vi "SCS Main.vi"() -> ()   [LabVIEW 2016]
doc: "Use this template to build a simple state machine design pattern. Each state executes code and determines which state to transition to."
uses:
  controls/SCS State.ctl
  controls/SCS Data.ctl
panel:
  in  "Solar Cell Stand Control":T1(tab)
  in  "NI Elvis Board":tag
  in  "Start Voltage, V:":dbl caption="MOSFET Control Voltage Range, V:"
  in  "Stop Voltage, V:":dbl=-10.0
  in  "Step Voltage, V:":dbl=0.1
  in  "Measurement pause, ms:":u32=250
  in  "Area of Solar Cell, m^2:":dbl=0.1
  in  "Light Intensity/ Irradiance, W/m^2:":dbl(knob)=600.0 scale=0.0..1200.0
  in  "Data from file":bool
  in  "Measure I-V Curve":bool
  out "Progress":u8(slide) max=100 scale=0.0..100.0
  out "Current (Amps) vs Voltage (Volts)":cluster{"voltage":dbl[], "current":dbl[]}(graph)
  in  "Voltage Data":path=path "E:/UPWORK/solar/labview/003/SolarCellStand/Sample Data/voltage - foward - bias - 001.lvm" caption="File Name"
  in  "Current Data":path=path "E:/UPWORK/solar/labview/003/SolarCellStand/Sample Data/current - foward - bias - 001.lvm" caption="File Name"
  in  "Calculate Solar Cell Parameters":bool
  out "Short Circuit Current Isc, A:":dbl format="%.5f"
  out "Open Circuit Voltage Voc, V:":dbl format="%.5f"
  out "Efficiency, %:":dbl format="%.5f"
  out "Fill Factor:":dbl format="%.5f"
  out "Pmax, W:":dbl format="%.5f"
  out "Voltage at Pmax, V:":dbl format="%.5f"
  out "Current at Pmax, A:":dbl format="%.5f"
  out "Current and Power vs. Voltage":cluster{"voltage":dbl[], "current":dbl[]}[](graph)=[{"voltage"=[0.00134, 0.011411, 0.025834, 0.043904, 0.055853, 0.075347, 0.099155, 0.125663, 0.165263, 0.217428, 0.267874, 0.315752, 0.36725, 0.425099, 0.474937, 0.530085, 0.588472, 0.643221, 0.694358, 0.754622, 0.812053, 0.873564, 0.938448, 0.995444, 1.055319, 1.116484, 1.181096, 1.242979, 1.310054, 1.384923, 1.457974, 1.528483, 1.591961, 1.655914, 1.723383, 1.78537, 1.841803, 1.874735, 1.918172, 1.968127, 2.017264, 2.064175, 2.116398, 2.158177, 2.191225, 2.218755, 2.24048, 2.261856, 2.280808, 2.297463, 2.312474, 2.325391, 2.338537, 2.350645, 2.362017, 2.372641, 2.381227, 2.390448, 2.39921, 2.407016, 2.414358, 2.421423, 2.428593, 2.435115, 2.441853, 2.447216, 2.45325, 2.459011, 2.464522, 2.470157, 2.474042, 2.47733, 2.481663, 2.486527, 2.491175, 2.496801, 2.501739, 2.507229, 2.511954, 2.515881, 2.519776, 2.523798, 2.526966, 2.530482, 2.534179, 2.537454, 2.540996, 2.544249, 2.547457, 2.550411, 2.553712, 2.556938, 2.559943, 2.562754, 2.565624, 2.568656, 2.571368, 2.573971, 2.576844, 2.579394, 2.581922, 2.584569, 2.58696, 2.589667, 2.592003, 2.594428, 2.596938, 2.59895, 2.601485, 2.603775, 2.606028, 2.608198, 2.610307, 2.6125, 2.614489, 2.616517, 2.618693, 2.620546, 2.622788, 2.624713, 2.626775, 2.628652, 2.630374, 2.632358, 2.634291, 2.635909, 2.637872, 2.639706, 2.6416, 2.64327, 2.64507, 2.646937, 2.64855, 2.650292, 2.651969, 2.653556, 2.655158, 2.656701, 2.658523, 2.66009, 2.661507, 2.663332, 2.664731, 2.666314, 2.667904, 2.669272, 2.67096, 2.672271, 2.67381, 2.675234, 2.676598, 2.67819, 2.679489, 2.681023, 2.682384, 2.683646, 2.68527, 2.686444, 2.688037, 2.689359, 2.69057, 2.692017, 2.693188, 2.694379, 2.695854, 2.697093, 2.698419, 2.699635, 2.700981, 2.702147, 2.703366, 2.704606, 2.705739, 2.707068, 2.708254, 2.70947, 2.710647, 2.711858, 2.713057, 2.714301, 2.71546, 2.716741, 2.717737, 2.719024, 2.720152, 2.72107, 2.722252, 2.723341, 2.724516, 2.725631, 2.726557, 2.727808, 2.728738, 2.72989, 2.731069, 2.732, 2.733089, 2.734104, 2.73519, 2.736257, 2.737217, 2.738296, 2.739307, 2.740423, 2.741454, 2.742348, 2.743357, 2.744268, 2.745417, 2.746408, 2.747273, 2.74838, 2.749326, 2.750382, 2.751351, 2.752211, 2.753257, 2.754209, 2.755152, 2.756018, 2.756854, 2.757837, 2.758826, 2.759727, 2.760683, 2.761421, 2.76238, 2.763236, 2.764109, 2.764945, 2.76579, 2.76688, 2.767667, 2.768646, 2.769522, 2.770365, 2.771362, 2.772145, 2.773009, 2.7739, 2.774781, 2.775641, 2.776447, 2.777355, 2.778196, 2.778952, 2.779808], "current"=[0.11683, 0.116793, 0.116696, 0.116612, 0.116353, 0.116156, 0.115983, 0.115806, 0.115674, 0.115608, 0.115475, 0.115277, 0.115048, 0.114847, 0.114559, 0.114304, 0.114054, 0.113759, 0.113435, 0.11314, 0.112824, 0.112487, 0.112162, 0.111794, 0.111412, 0.111022, 0.11061, 0.110173, 0.109698, 0.109199, 0.108699, 0.1082, 0.107699, 0.107197, 0.106697, 0.106198, 0.105698, 0.105198, 0.104695, 0.104194, 0.103695, 0.103195, 0.102695, 0.102193, 0.101693, 0.101194, 0.100694, 0.10019, 0.09969, 0.09919, 0.098688, 0.098188, 0.097687, 0.097188, 0.096685, 0.096185, 0.095685, 0.095182, 0.094683, 0.094182, 0.093684, 0.093181, 0.092681, 0.09218, 0.091678, 0.091179, 0.090679, 0.090175, 0.089677, 0.089173, 0.088675, 0.088175, 0.087671, 0.087173, 0.086673, 0.086171, 0.085671, 0.085168, 0.08467, 0.08417, 0.083668, 0.083169, 0.082665, 0.082166, 0.081662, 0.081164, 0.080665, 0.080162, 0.079663, 0.079161, 0.07866, 0.078158, 0.077659, 0.077157, 0.076657, 0.076154, 0.075655, 0.075152, 0.074654, 0.074151, 0.073652, 0.07315, 0.07265, 0.072148, 0.071649, 0.071146, 0.070648, 0.070145, 0.069642, 0.069142, 0.068641, 0.068141, 0.067638, 0.067141, 0.066638, 0.066136, 0.065636, 0.065134, 0.064635, 0.064133, 0.063635, 0.063132, 0.062629, 0.06213, 0.061629, 0.061126, 0.060626, 0.060125, 0.059626, 0.059125, 0.058622, 0.058124, 0.057621, 0.057119, 0.056621, 0.056118, 0.055616, 0.055117, 0.054616, 0.054112, 0.053614, 0.053113, 0.05261, 0.052112, 0.051611, 0.051108, 0.05061, 0.050108, 0.049607, 0.049108, 0.048606, 0.048102, 0.047606, 0.047103, 0.046601, 0.046103, 0.045601, 0.045099, 0.044597, 0.044099, 0.043596, 0.043094, 0.042597, 0.042095, 0.041591, 0.041095, 0.040592, 0.040089, 0.039591, 0.03909, 0.038588, 0.038087, 0.037589, 0.037087, 0.036585, 0.036086, 0.035586, 0.035083, 0.034584, 0.034083, 0.033583, 0.033083, 0.032581, 0.03208, 0.031582, 0.03108, 0.030583, 0.030082, 0.029579, 0.02908, 0.02858, 0.028078, 0.02758, 0.02708, 0.026582, 0.026079, 0.025578, 0.025081, 0.02458, 0.02408, 0.02358, 0.023082, 0.02258, 0.022079, 0.021581, 0.021081, 0.020581, 0.020081, 0.019536, 0.019036, 0.018535, 0.018034, 0.017533, 0.017033, 0.016532, 0.016031, 0.01553, 0.01503, 0.014529, 0.014028, 0.013528, 0.013027, 0.012526, 0.012026, 0.011525, 0.011024, 0.010524, 0.010023, 0.009523, 0.009022, 0.008521, 0.00802, 0.007519, 0.007018, 0.006517, 0.006016, 0.005515, 0.005015, 0.004514, 0.004013, 0.003512, 0.003012, 0.002512, 0.002012, 0.001507, 0.001006, 0.000505]}, {"voltage"=[0.00134, 0.011411, 0.025834, 0.043904, 0.055853, 0.075347, 0.099155, 0.125663, 0.165263, 0.217428, 0.267874, 0.315752, 0.36725, 0.425099, 0.474937, 0.530085, 0.588472, 0.643221, 0.694358, 0.754622, 0.812053, 0.873564, 0.938448, 0.995444, 1.055319, 1.116484, 1.181096, 1.242979, 1.310054, 1.384923, 1.457974, 1.528483, 1.591961, 1.655914, 1.723383, 1.78537, 1.841803, 1.874735, 1.918172, 1.968127, 2.017264, 2.064175, 2.116398, 2.158177, 2.191225, 2.218755, 2.24048, 2.261856, 2.280808, 2.297463, 2.312474, 2.325391, 2.338537, 2.350645, 2.362017, 2.372641, 2.381227, 2.390448, 2.39921, 2.407016, 2.414358, 2.421423, 2.428593, 2.435115, 2.441853, 2.447216, 2.45325, 2.459011, 2.464522, 2.470157, 2.474042, 2.47733, 2.481663, 2.486527, 2.491175, 2.496801, 2.501739, 2.507229, 2.511954, 2.515881, 2.519776, 2.523798, 2.526966, 2.530482, 2.534179, 2.537454, 2.540996, 2.544249, 2.547457, 2.550411, 2.553712, 2.556938, 2.559943, 2.562754, 2.565624, 2.568656, 2.571368, 2.573971, 2.576844, 2.579394, 2.581922, 2.584569, 2.58696, 2.589667, 2.592003, 2.594428, 2.596938, 2.59895, 2.601485, 2.603775, 2.606028, 2.608198, 2.610307, 2.6125, 2.614489, 2.616517, 2.618693, 2.620546, 2.622788, 2.624713, 2.626775, 2.628652, 2.630374, 2.632358, 2.634291, 2.635909, 2.637872, 2.639706, 2.6416, 2.64327, 2.64507, 2.646937, 2.64855, 2.650292, 2.651969, 2.653556, 2.655158, 2.656701, 2.658523, 2.66009, 2.661507, 2.663332, 2.664731, 2.666314, 2.667904, 2.669272, 2.67096, 2.672271, 2.67381, 2.675234, 2.676598, 2.67819, 2.679489, 2.681023, 2.682384, 2.683646, 2.68527, 2.686444, 2.688037, 2.689359, 2.69057, 2.692017, 2.693188, 2.694379, 2.695854, 2.697093, 2.698419, 2.699635, 2.700981, 2.702147, 2.703366, 2.704606, 2.705739, 2.707068, 2.708254, 2.70947, 2.710647, 2.711858, 2.713057, 2.714301, 2.71546, 2.716741, 2.717737, 2.719024, 2.720152, 2.72107, 2.722252, 2.723341, 2.724516, 2.725631, 2.726557, 2.727808, 2.728738, 2.72989, 2.731069, 2.732, 2.733089, 2.734104, 2.73519, 2.736257, 2.737217, 2.738296, 2.739307, 2.740423, 2.741454, 2.742348, 2.743357, 2.744268, 2.745417, 2.746408, 2.747273, 2.74838, 2.749326, 2.750382, 2.751351, 2.752211, 2.753257, 2.754209, 2.755152, 2.756018, 2.756854, 2.757837, 2.758826, 2.759727, 2.760683, 2.761421, 2.76238, 2.763236, 2.764109, 2.764945, 2.76579, 2.76688, 2.767667, 2.768646, 2.769522, 2.770365, 2.771362, 2.772145, 2.773009, 2.7739, 2.774781, 2.775641, 2.776447, 2.777355, 2.778196, 2.778952, 2.779808], "current"=[0.0001565522, 0.0013327249229999998, 0.0030147244639999998, 0.0051197332479999995, 0.0064986641089999995, 0.008752006132, 0.011500294365, 0.014552529378000001, 0.019116632262, 0.025136416224, 0.030932750149999997, 0.036398943304, 0.042251378, 0.048821344853, 0.054408307782999994, 0.06059083584, 0.067117585488, 0.073172177739, 0.07876449972999999, 0.08537793308000001, 0.091619067672, 0.098264593668, 0.10525820457599999, 0.111284666536, 0.11757520042799999, 0.123954286648, 0.13064102855999998, 0.136942725367, 0.14371030369200002, 0.151232206677, 0.15848031582600003, 0.1653818606, 0.171452607739, 0.17750901305800001, 0.183879795951, 0.18960272326, 0.194674893494, 0.19721837253, 0.20082301753999998, 0.20506702463799997, 0.20918019047999997, 0.213012539125, 0.21734349260999997, 0.220550582161, 0.22283224392500003, 0.22452469346999998, 0.22560289311999998, 0.22661535264, 0.22737374952, 0.22788535497, 0.22821343411199999, 0.22832549150800002, 0.228444663919, 0.22845448626, 0.22837161364499997, 0.228212474585, 0.22784770549500002, 0.227527621536, 0.22716440043000002, 0.226697580912, 0.226186714872, 0.22563061656299999, 0.22508442783299998, 0.2244689007, 0.22386419933399998, 0.223134707664, 0.22245825675, 0.221741316925, 0.22101093939400002, 0.220271310161, 0.21938567435, 0.21843857275, 0.217569876873, 0.21675801817100002, 0.21591761077500002, 0.215151838971, 0.214326481869, 0.213535679472, 0.21268714517999998, 0.21176170376999998, 0.210824618368, 0.20990175586200002, 0.20889164439, 0.20791958401200003, 0.20694612549799998, 0.205949916456, 0.20496944233999997, 0.20395208833800002, 0.202938066991, 0.201893085171, 0.20087498591999997, 0.19984516020400003, 0.198802613437, 0.19773441037800002, 0.196673038968, 0.19561342902399997, 0.19453684604000002, 0.19343906859199997, 0.19237171197599998, 0.191264644494, 0.190163719144, 0.18906122235000003, 0.18794264400000002, 0.186839294716, 0.18571442294700002, 0.18458317448800002, 0.18346847582400003, 0.18230334774999998, 0.18117261836999998, 0.18003021105, 0.17888036794799997, 0.17772521991799997, 0.17655594486600001, 0.1754058625, 0.174224317982, 0.173045968312, 0.171880533748, 0.170686643164, 0.16952390237999998, 0.16833071882899997, 0.167154827125, 0.16595205806399999, 0.16473769324600002, 0.16354840254, 0.16234872003900003, 0.161122573534, 0.159923627872, 0.15871232324999998, 0.15750804159999998, 0.15628333874999997, 0.15505929354, 0.153850566188, 0.15261209955000002, 0.151382028748, 0.15015713674899997, 0.148912255608, 0.147669267328, 0.146429389017, 0.145197892168, 0.14394279008, 0.142694036298, 0.141457552516, 0.14019149791, 0.13894695516799999, 0.137693193344, 0.136421153376, 0.1351772856, 0.13390215526799998, 0.13263969267, 0.131375391272, 0.130098722388, 0.12882629537999998, 0.127559753334, 0.126284226369, 0.12500177678399998, 0.12372413153799999, 0.12245099727000001, 0.12115593795599999, 0.11987838608899999, 0.118598042541, 0.11729808972000001, 0.11600978059799999, 0.11472172923600002, 0.113419884005, 0.11212326371400001, 0.110837036835, 0.109534224048, 0.10822566751499998, 0.10693453877100001, 0.10562692623, 0.10431748720799999, 0.10301032872200001, 0.10170602327099999, 0.10039703091600001, 0.09908147259000001, 0.09777393442, 0.096461084142, 0.09514011421400001, 0.093828363288, 0.092511520983, 0.09119329318000001, 0.089877942503, 0.088546589197, 0.08722628991999999, 0.085907840464, 0.08457085560000001, 0.08325463291600001, 0.08192354396200001, 0.080588458764, 0.07926134948, 0.07792499906000001, 0.07659139302399999, 0.07525859404, 0.07392542120000001, 0.072597276158, 0.07124782800000001, 0.069906950442, 0.06857406242399999, 0.0672309702, 0.06588906856, 0.06454357686, 0.063205348272, 0.061853552060000004, 0.060505799417, 0.059163318774, 0.05781143818799999, 0.056461030417, 0.055107645708, 0.05363446651200001, 0.052280622688, 0.050920705054999994, 0.04956428492000001, 0.048203932758, 0.046847256606, 0.045485334732000005, 0.044120694541, 0.04275808121, 0.04139576127, 0.040029603408, 0.038661420504, 0.037294720912, 0.035926342599, 0.034557054476, 0.033188476902, 0.031816871575, 0.030441905104, 0.02907128712, 0.027695914428000002, 0.026322610007, 0.024945333790000003, 0.02356729659, 0.0221903776, 0.020810088172999997, 0.019430357627999998, 0.018048974874, 0.01666651584, 0.015284061429999999, 0.013902307175000002, 0.012517362625999999, 0.011131660699999999, 0.009745030872, 0.008360230691999999, 0.006974434864, 0.00558803826, 0.004186741372, 0.0027956257119999997, 0.0014038030400000002]}]
  in  "Exit":bool
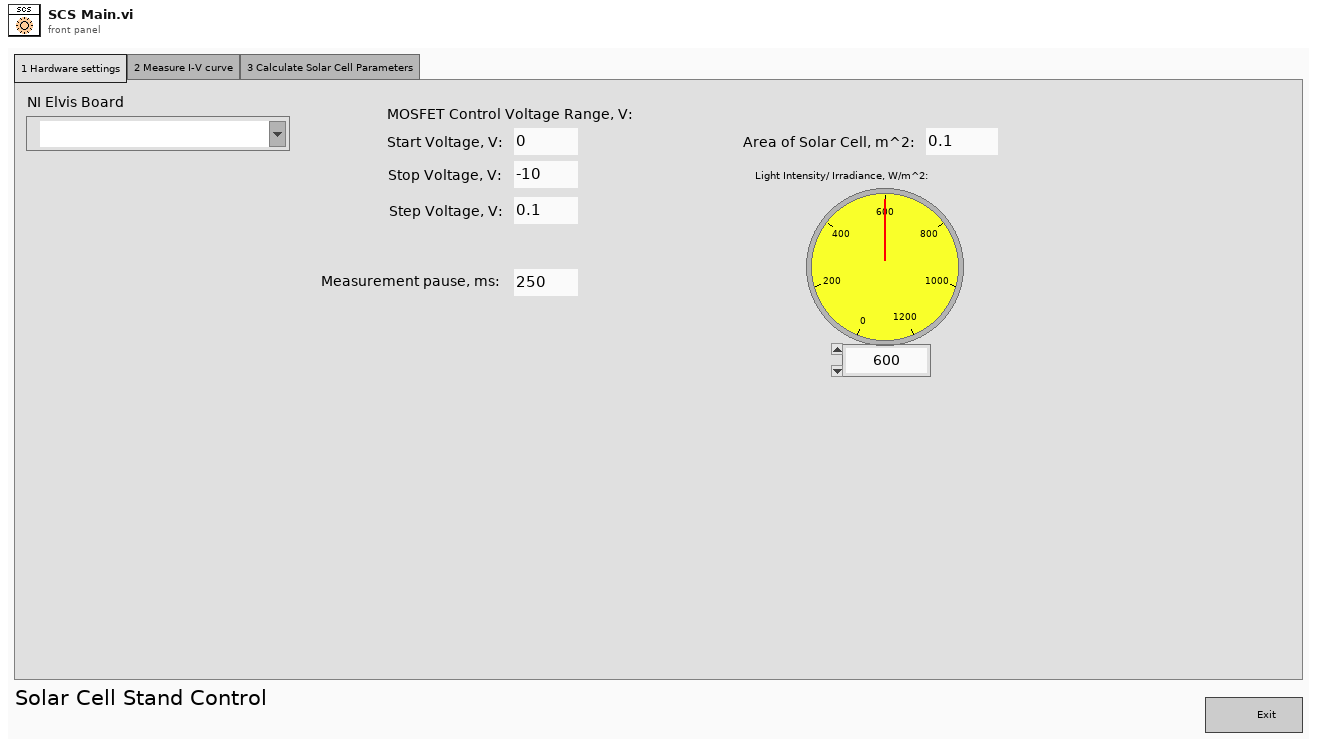
[diagram p1: front panel]
types:
  T1 = enum32{"1 Hardware settings", "2 Measure I-V curve", "3 Calculate Solar Cell Parameters"}
  T2 = typedef "SCS Data.ctl" = cluster{"Done":bool, "Current Array":dbl[], "Voltage Array":dbl[]}
  T3 = typedef "SCS State.ctl" = enum16{"Initialize", "Wait for Event", "Measure I-V curve", "Calculate Solar Cell Parameters", "Exit"}
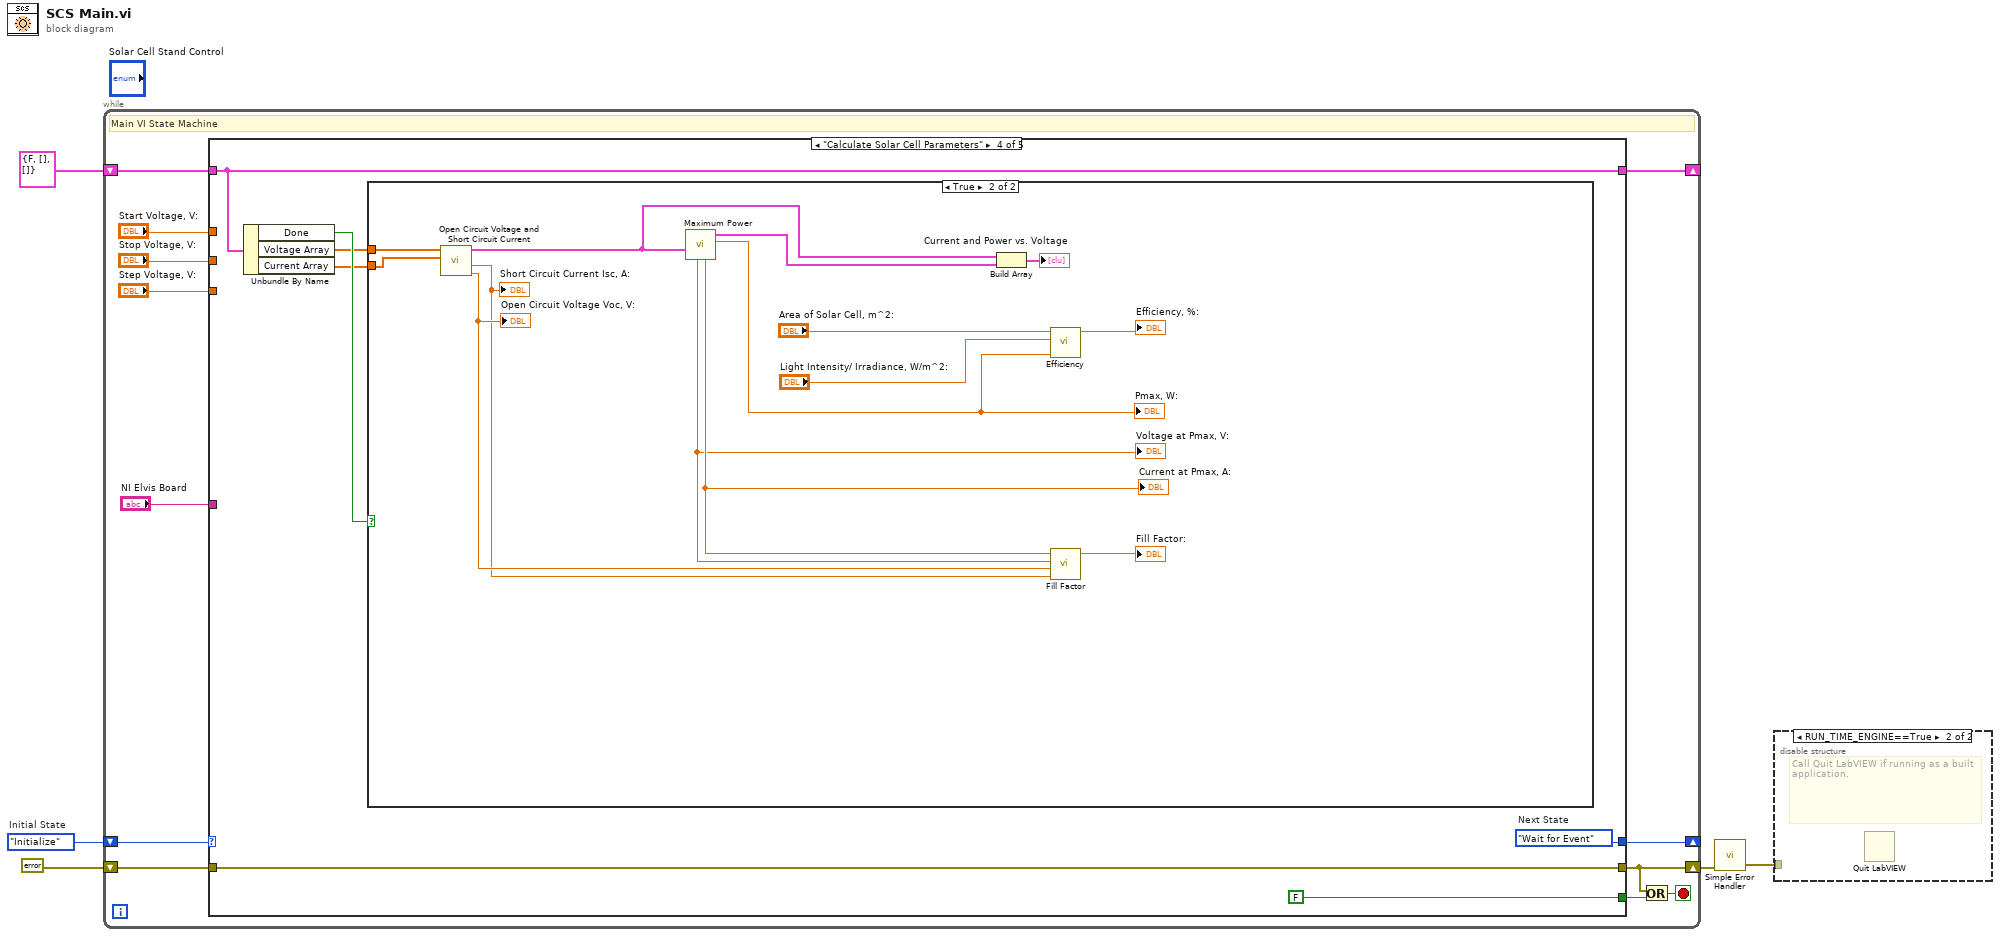
[diagram p0: block diagram]
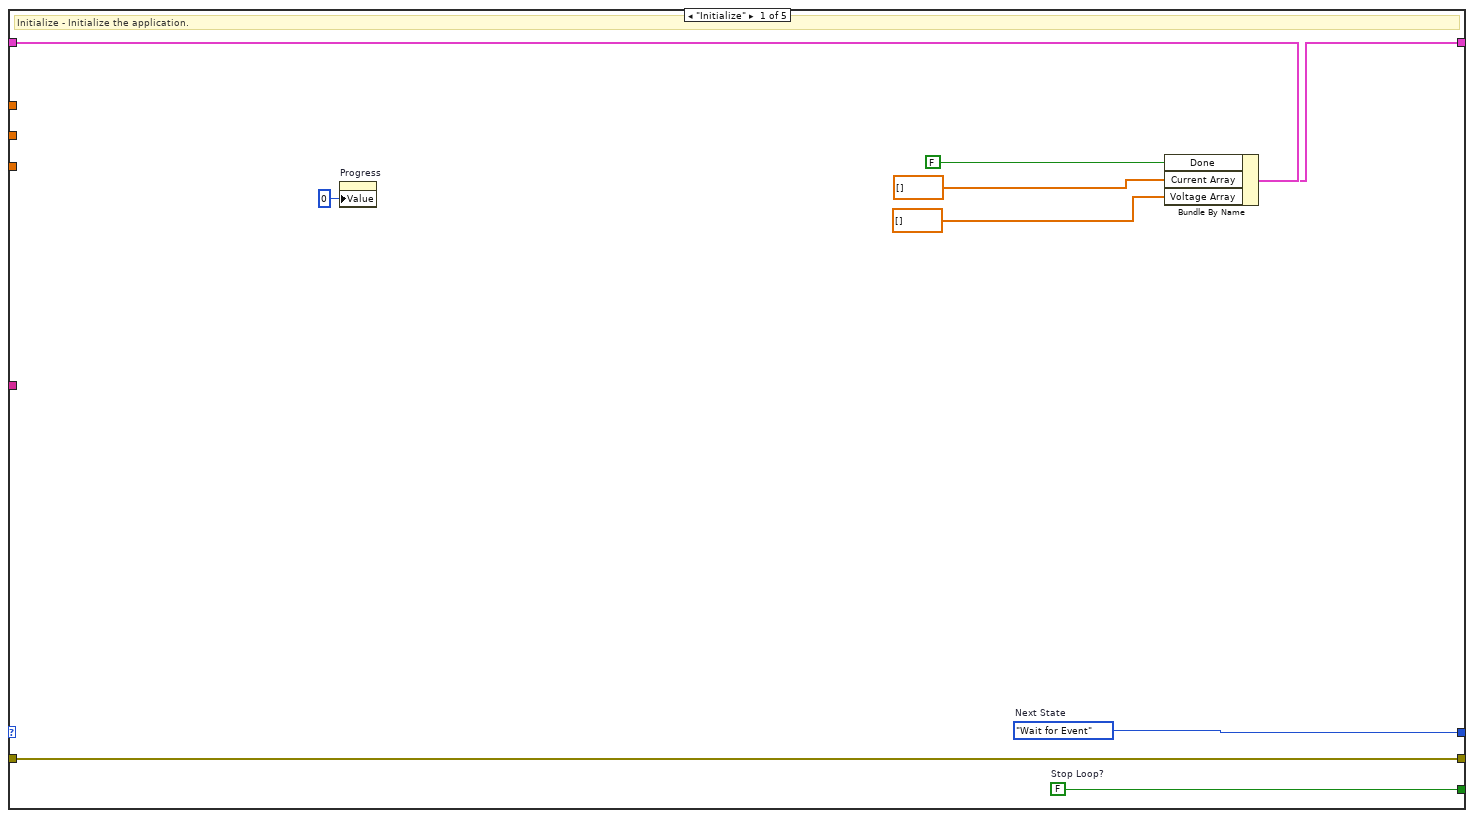
[diagram p3: hidden frame]
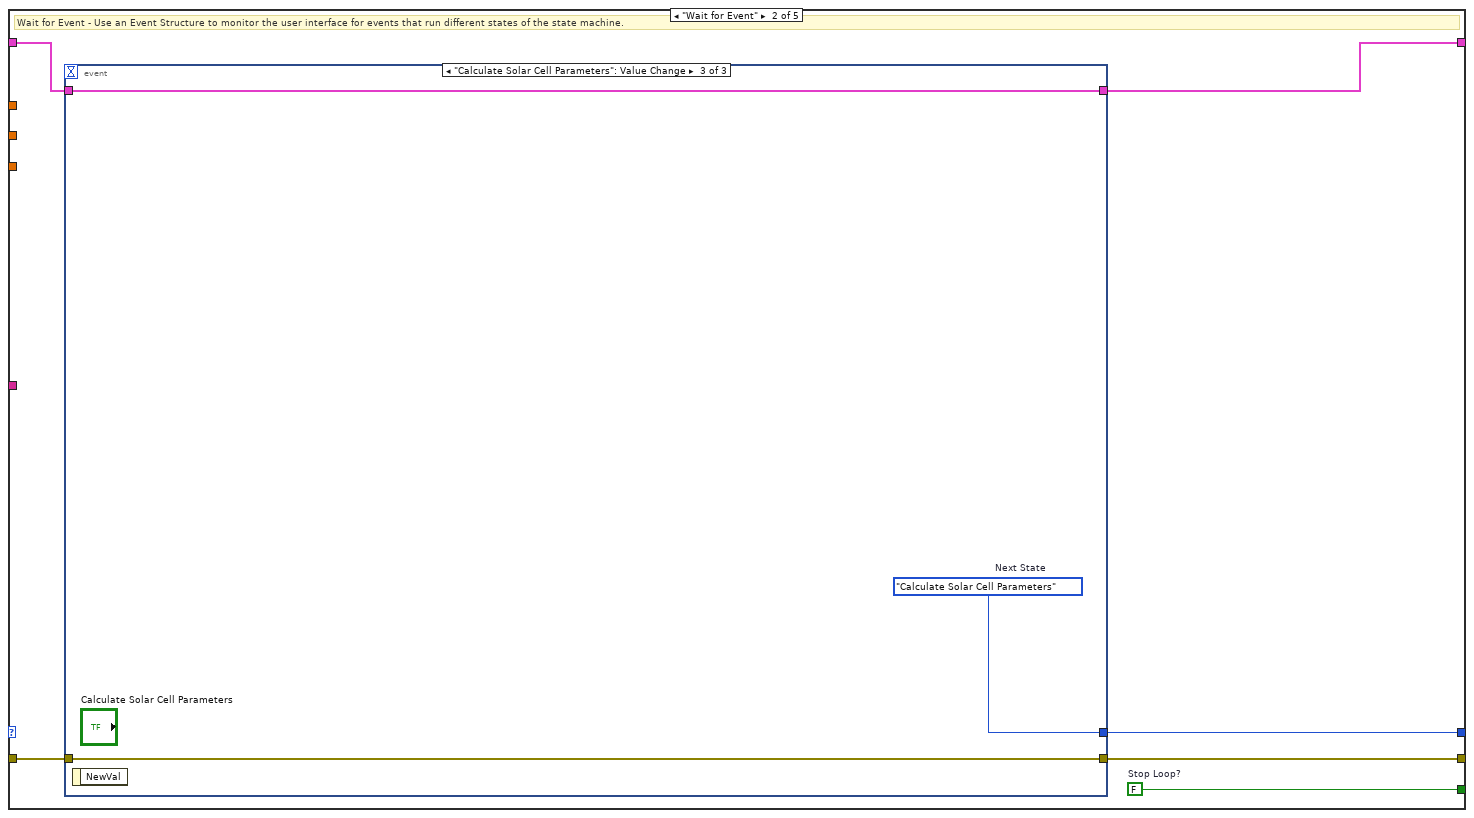
[diagram p4: hidden frame]
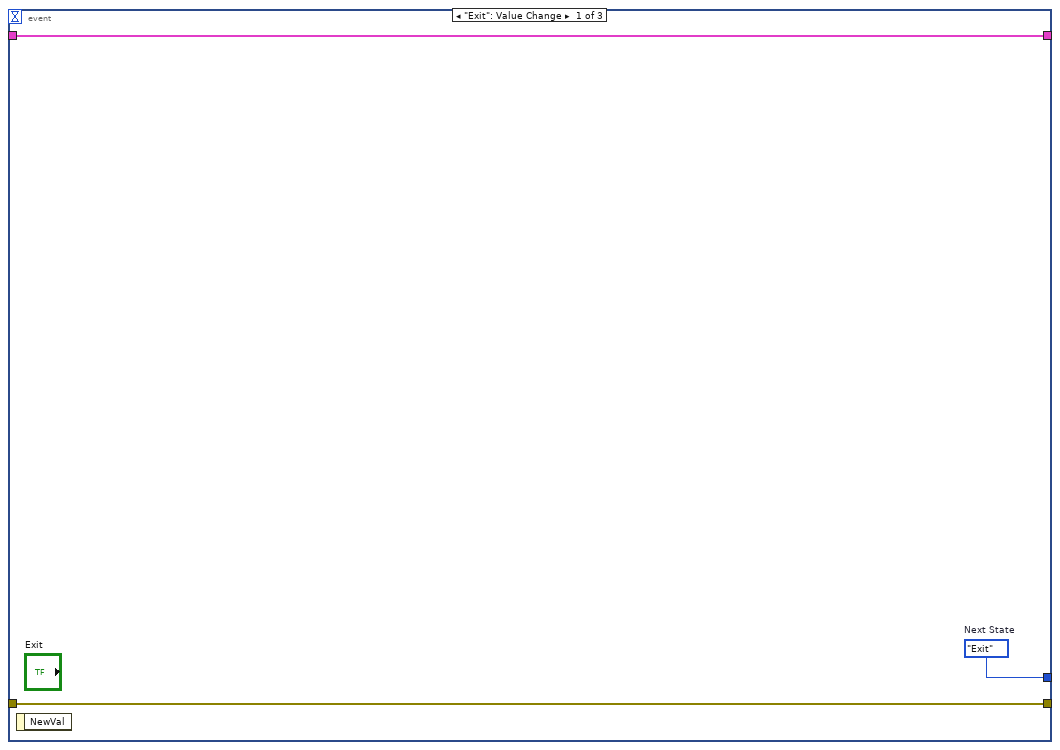
[diagram p5: hidden frame]
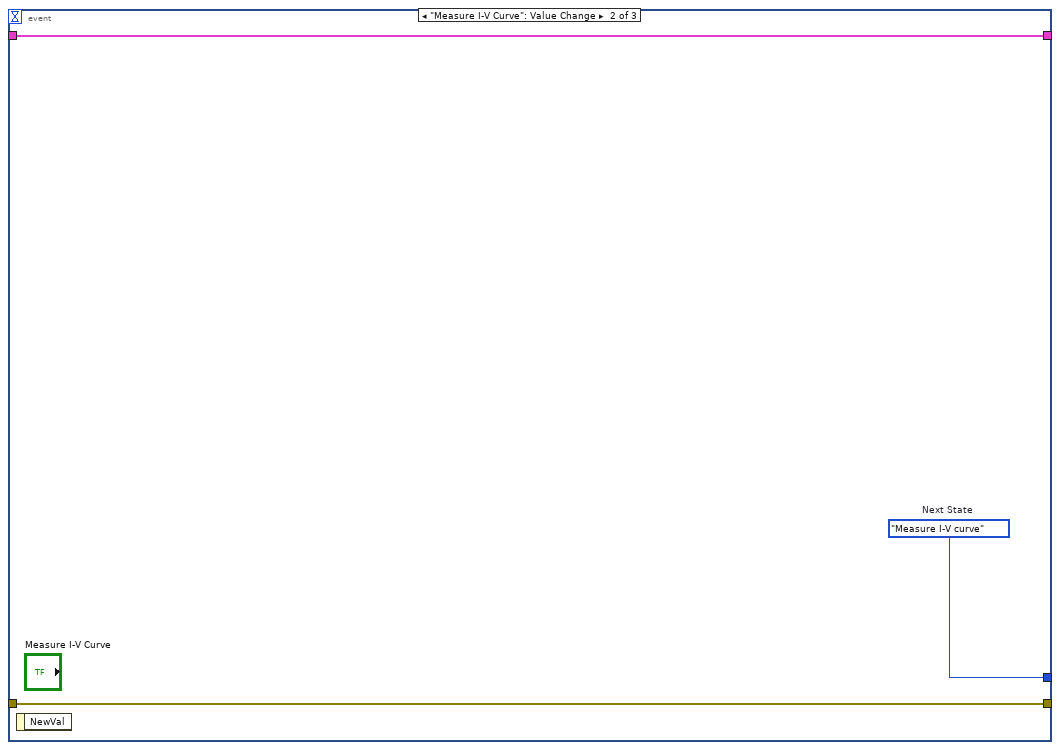
[diagram p6: hidden frame]
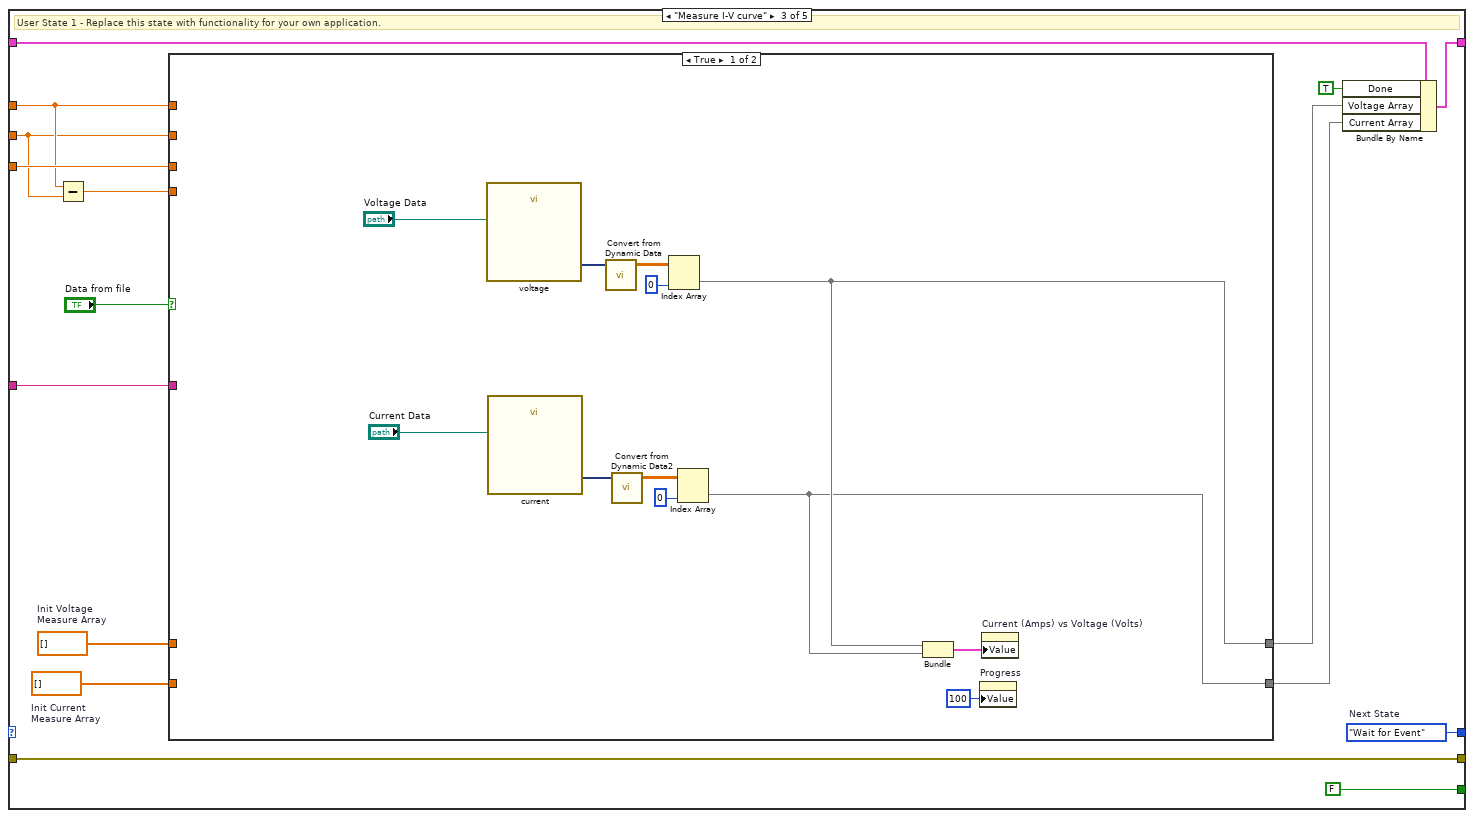
[diagram p7: hidden frame]
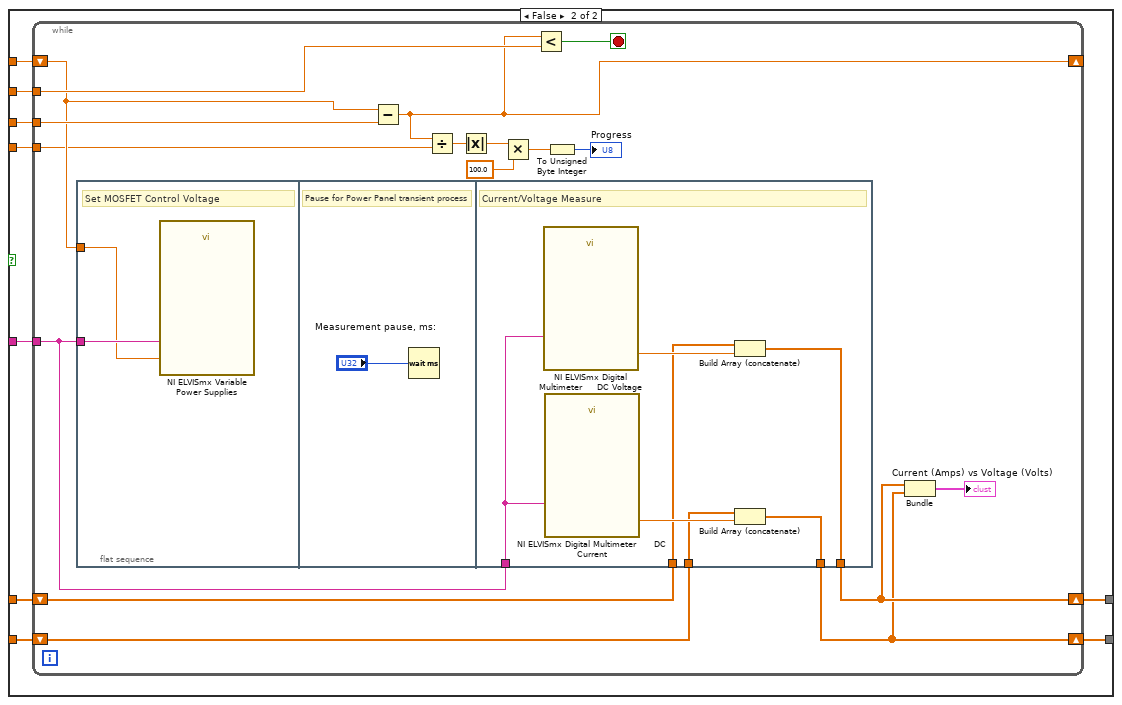
[diagram p8: hidden frame]
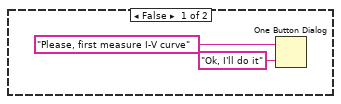
[diagram p9: hidden frame]
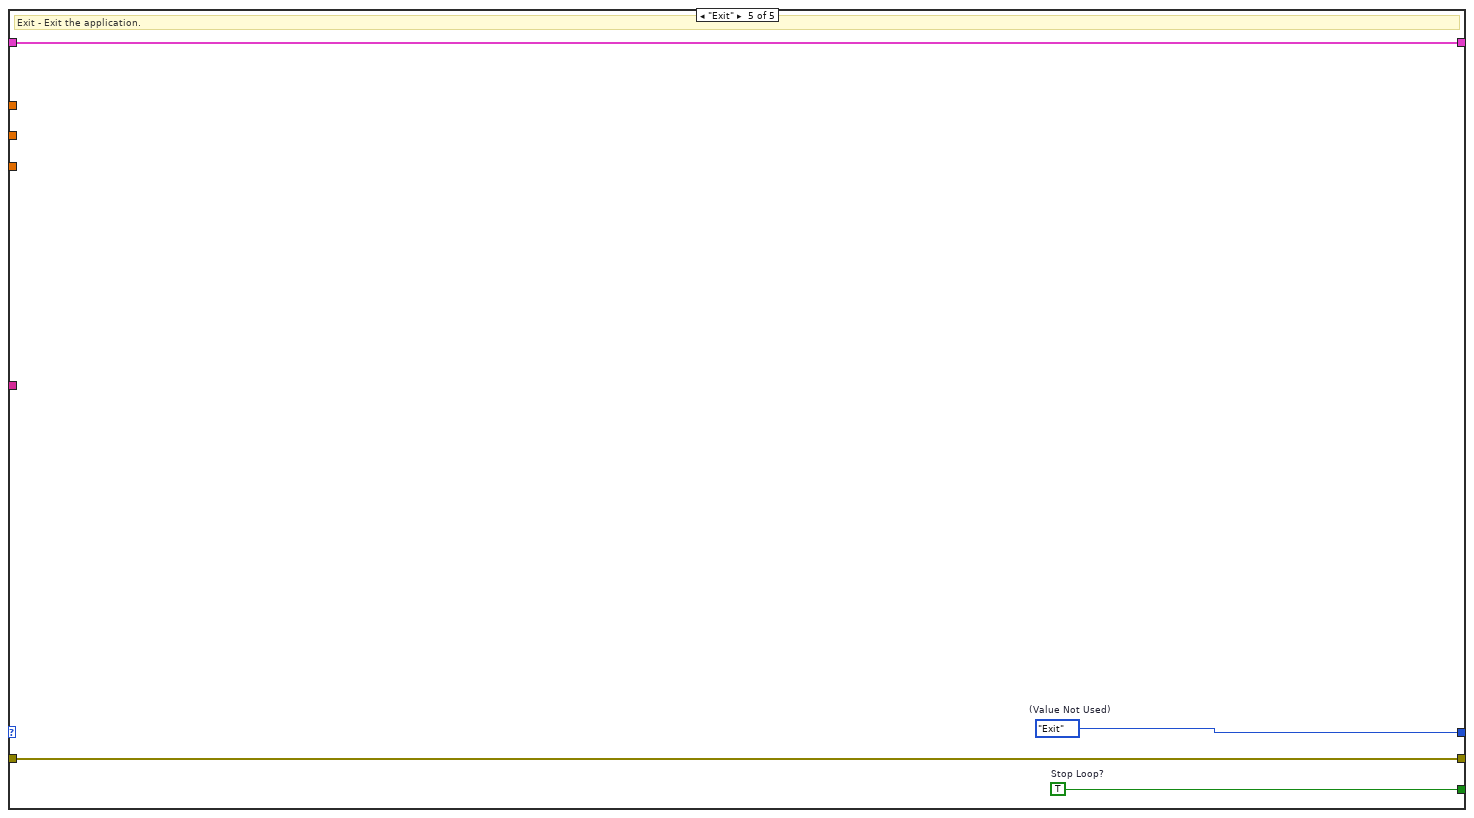
[diagram p10: hidden frame]
diagram:
  w5 = SCS_State."Initialize"  # Initial State
  n1 = while {
    shift-right: [w16] -> _
    shift-left: w5 -> [w17]
    shift-right: [w14] -> _
    shift-left: T2 {"Done"=FALSE, "Current Array"=[], "Voltage Array"=[]} ("Data") -> [w15]
    shift-right: [w10] -> w2
    shift-left: errorcluster {"status"=FALSE, "code"=0, "source"=""} ("error constant") -> [w13]
    stop <- w11 stop-if-true
    # "Main VI State Machine"
    n2 = case shown="\"Calculate Solar Cell Parameters\"" w17 {
      tunnel: [w26 w32 w57 w112 w132] -> w16
      tunnel: [w25 w31 FALSE ("Stop Loop?") FALSE ("Stop Loop?") w130] -> w12
      tunnel: w15 -> [w24 w30 w47 w109 w131]
      tunnel: [w23 w29 w46 w109 w131] -> w14
      tunnel: w13 -> [w21 w28 w55 w110 w129]
      tunnel: [w21 w27 w55 w110 w129] -> w10
      tunnel: "Start Voltage, V:" -> [_ _ w50 _ _]
      tunnel: "Stop Voltage, V:" -> [_ _ w49 _ _]
      tunnel: "Step Voltage, V:" -> [_ _ w52 _ _]
      tunnel: "NI Elvis Board" -> [_ _ w51 _ _]
      frame "Initialize" {
        w25 = FALSE  # Stop Loop?
        w26 = SCS_State."Wait for Event"  # Next State
        # "Initialize - Initialize the application."
        n3 = property on="Progress" class="Slide (strict)"("Value"=u8 0 ("Progress")) -> ()  [unwired: 2 in, 2 out]
        n4 = Bundle By Name(cluster=w24, "Done"=FALSE ("Replace_Me_Boolean"), "Current Array"=dbl[] [], "Voltage Array"=dbl[] []) -> (w23:T2)
      }
      frame "Wait for Event" {
        w31 = FALSE  # Stop Loop?
        # "Wait for Event - Use an Event Structure to monitor the user interface for events that run different states of the state machine."
        n5 = event shown="[2] \"Calculate Solar Cell Parameters\": Value Change" {
          selector: _ -> [_ _ _]
          dyn-events: _ -> [_ _ _]
          timeout: _ -> [_ _ _]
          tunnel: [w35 w38 w41] -> w32
          tunnel: w30 -> [w34 w36 w39]
          tunnel: [w34 w36 w39] -> w29
          tunnel: w28 -> [w33 w37 w40]
          tunnel: [w33 w37 w40] -> w27
          event "Exit": Value Change {
            w35 = SCS_State."Exit"  # Next State
            n6 = event-data() -> ()  [unwired: 1 in, 1 out]
          }
          event "Measure I-V Curve": Value Change {
            w38 = SCS_State."Measure I-V curve"  # Next State
            n7 = event-data() -> ()  [unwired: 1 in, 1 out]
          }
          event "Calculate Solar Cell Parameters": Value Change {
            w41 = SCS_State."Calculate Solar Cell Parameters"  # Next State
            n8 = event-data() -> ()  [unwired: 1 in, 1 out]
          }
        }
      }
      frame "Measure I-V curve" {
        w53 = dbl[] []  # Init Current  Measure Array
        w54 = dbl[] []  # Init Voltage Measure Array
        w57 = SCS_State."Wait for Event"  # Next State
        # "User State 1 - Replace this state with functionality for your own application."
        n9 = Subtract(x=w50, y=w49) -> (x-y=w48:dbl)
        n10 = case shown="True" "Data from file" {
          tunnel: w54 -> [_ w78]
          tunnel: w53 -> [_ w77]
          tunnel: w52 -> [_ w76]
          tunnel: w51 -> [_ w75]
          tunnel: w50 -> [_ w74]
          tunnel: w49 -> [_ w73]
          tunnel: w48 -> [_ w72]
          tunnel: [w61 w71] -> w44
          tunnel: [w60 w70] -> w43
          frame True {
            n11 = call "voltage"("File Name"="Voltage Data") -> ("Signals"=w67:dynamicdata)  [unwired: 3 in, 7 out]
            n12 = call "current"("File Name"="Current Data") -> ("Signals"=w66:dynamicdata)  [unwired: 3 in, 7 out]
            n13 = call "Convert from Dynamic Data"("Dynamic Data Type"=w67) -> ("Array"=w65:dbl[][])  [unwired: 3 out]
            n14 = call "Convert from Dynamic Data2"("Dynamic Data Type"=w66) -> ("Array"=w64:dbl[][])  [unwired: 3 out]
            n15 = Index Array(array=w65, index (col)=0 ("disabled index (col)")) -> (element=w61:dbl[])  [unwired: 1 in]
            n16 = Index Array(array=w64, index (col)=0 ("disabled index (col)")) -> (element=w60:dbl[])  [unwired: 1 in]
            n17 = Bundle("Array"=w61, "Array"=w60) -> (w59:cluster{"Array":dbl[], "Array":dbl[]})  [unwired: 1 out]
            n18 = property on="Progress" class="Slide (strict)"("Value"=u8 100 ("Progress")) -> ()  [unwired: 2 in, 2 out]
            n19 = property on="Current (Amps) vs Voltage (Volts)" class="XYGraph (strict)"("Value"=w59) -> ()  [unwired: 2 in, 2 out]
          }
          frame False {
            n20 = while {
              tunnel: w73 -> [w94]
              tunnel: w76 -> [w95]
              shift-right: [w88] -> _
              shift-left: w74 -> [w92]
              shift-right: [w80] -> w71
              shift-left: w78 -> [w90]
              shift-right: [w79] -> w70
              shift-left: w77 -> [w89]
              tunnel: w75 -> [w91]
              tunnel: w72 -> [w87]
              stop <- w93 stop-if-true
              n21 = flat-sequence {
                tunnel: w92 -> [w96]
                tunnel: w91 -> [w97]
                tunnel: w91 -> [w103]
                tunnel: w90 -> [w102]
                tunnel: w89 -> [w101]
                tunnel: [w100] -> w80
                tunnel: [w99] -> w79
                frame #0 {
                  # "Set MOSFET Control Voltage"
                  n22 = call "NI ELVISmx Variable Power Supplies"("Device Name"=w97, "Supply- (V)"=w96) -> ()  [unwired: 15 in, 3 out]
                }
                frame #1 {
                  # "Pause for Power Panel transient process"
                  n23 = Wait (ms)(milliseconds to wait="Measurement pause, ms:") -> ()  [unwired: 1 out]
                }
                frame #2 {
                  # "Current/Voltage Measure"
                  n24 = call "NI ELVISmx Digital Multimeter     DC Voltage"("Device Name"=w103) -> ("Measurement"=w105:dbl)  [unwired: 16 in, 2 out]
                  n25 = call "NI ELVISmx Digital Multimeter      DC Current"("Device Name"=w103) -> ("Measurement"=w104:dbl)  [unwired: 16 in, 2 out]
                  n26 = Build Array (concatenate)(w102, w105) -> (w100:dbl[])
                  n27 = Build Array (concatenate)(w101, w104) -> (w99:dbl[])
                }
              }
              n28 = Subtract(x=w92, y=w95) -> (x-y=w88:dbl)
              n29 = Divide(x=w88, y=w87) -> (x/y=w86:dbl)
              n30 = Absolute Value(x=w86) -> (abs(x)=w85:dbl)
              n31 = Multiply(x=w85, y=100.0) -> (x*y=w83:dbl)
              n32 = Less?(x=w88, y=w94) -> (x < y?=w93:bool)
              n33 = To Unsigned Byte Integer(number=w83) -> (unsigned 8bit integer=→"Progress":u8)
              n34 = Bundle(w80, w79) -> (→"Current (Amps) vs Voltage (Volts)":cluster{dbl[], dbl[]})  [unwired: 1 out]
            }
          }
        }
        n35 = Bundle By Name(cluster=w47, "Done"=TRUE, "Voltage Array"=w44, "Current Array"=w43) -> (w46:T2)
      }
      frame "Calculate Solar Cell Parameters" {
        w112 = SCS_State."Wait for Event"  # Next State
        n36 = Unbundle By Name(w109) -> ("Done"=w108:bool, "Voltage Array"=w107:dbl[], "Current Array"=w106:dbl[])
        n37 = case shown="True" w108 {
          tunnel: w107 -> [_ w128]
          tunnel: w106 -> [_ w127]
          frame False {
            n38 = One Button Dialog(message="Please, first measure I-V curve", button name ("OK")="Ok, I'll do it") -> ()  [unwired: 1 out]
          }
          frame True {
            n39 = call "Open Circuit Voltage and Short Circuit Current.vi"("Current"=w127, "Voltage"=w128) -> ("Open Circuit Voltage"=w124:dbl, "Short Circuit Current"=w123:dbl, "Current (Amps) vs Voltage (Volts)"=w116:cluster{"voltage":dbl[], "current":dbl[]})  [unwired: 5 in, 2 out]
            "Short Circuit Current Isc, A:" <- w123
            "Open Circuit Voltage Voc, V:" <- w124
            n40 = call "Maximum Power.vi"("Current (Amps) vs Voltage (Volts)"=w116) -> ("Maximum Power"=w120:dbl, "Power (Watts) vs Voltage (Volts)"=w115:cluster{"voltage":dbl[], dbl[]}, "Current at Pmax"=w119:dbl, "Voltage at Pmax"=w118:dbl)  [unwired: 7 in]
            "Pmax, W:" <- w120
            "Voltage at Pmax, V:" <- w118
            "Current at Pmax, A:" <- w119
            n41 = Build Array(w116, w115) -> (→"Current and Power vs. Voltage":cluster{"voltage":dbl[], "current":dbl[]}[])
            n42 = call "Efficiency.vi"("Maximum Power"=w120, "Irradiance"="Light Intensity/ Irradiance, W/m^2:", "Area"="Area of Solar Cell, m^2:") -> ("Efficiency"=→"Efficiency, %:":dbl)  [unwired: 8 in]
            n43 = call "Fill Factor.vi"("Current at Short Circuit"=w123, "Voltage at Open Circuit"=w124, "Voltage at Max Power"=w118, "Current at Max Power"=w119) -> ("Fill factor"=→"Fill Factor:":dbl)  [unwired: 7 in]
          }
        }
      }
      frame "Exit" {
        w130 = TRUE  # Stop Loop?
        w132 = SCS_State."Exit"  # (Value Not Used)
        # "Exit - Exit the application."
      }
    }
    n44 = Or(x=w10, y=w12) -> (x .or. y?=w11:bool)
  }
  n45 = call <vilib>:"Simple Error Handler.vi"("error in (no error)"=w2) -> ("error out"=w1:errorcluster)  [unwired: 4 in, 4 out]
  n46 = disable-structure shown="RUN_TIME_ENGINE==True" {
    disable-tunnel: w1 -> [_ _]
    frame condition #0 (active) {
    }
    frame condition #1 {
      # "Call Quit LabVIEW if running as a built application."
      n47 = Quit LabVIEW() -> ()  [unwired: 1 in]
    }
  }
